vi "dl950_wave1.vi"() -> ()   [LabVIEW 2019]
uses:
  <instrlib>/Yokogawa DL950 Series/Public/Configure/Configure Module (Voltage).vi
  <instrlib>/Yokogawa DL950 Series/Public/Data/Read Waveform (Single).vi
  <instrlib>/Yokogawa DL950 Series/Yokogawa DL950 Series.lvlib
panel:
  in  "Channel (1: CH1)":u16(ring)=1 items=["", "CH1", "CH2", "CH3", "CH4", "CH5", "CH6", "CH7", "CH8", "CH9", "CH10", "CH11", "CH12", "CH13", "CH14", "CH15", "CH16"]
  in  "Vertical Coupling (1: DC)":i32(ring)=1 items=["AC", "DC", "Ground", "AC-RMS", "DC-RMS"]
  in  "Enable Calibration (F: No)":bool
  in  "Enable Auto Setup (T: Yes)":bool=TRUE
  in  "VISA resource name":refnum<visa-resource-name>
  in  "Source (1: CH1)":u16(ring)=1 items=["", "CH1", "CH2", "CH3", "CH4", "CH5", "CH6", "CH7", "CH8", "CH9", "CH10", "CH11", "CH12", "CH13", "CH14", "CH15", "CH16", "MATH1", "MATH2", "MATH3", "MATH4", "MATH5", "MATH6", "MATH7", "MATH8", "EVENT"]
  in  "Sub Channel (0: None)":i16(ring) items=["None", "SCH1", "SCH2", "SCH3", "SCH4", "SCH5", "SCH6", "SCH7", "SCH8", "SCH9", "SCH10", "SCH11", "SCH12", "SCH13", "SCH14", "SCH15", "SCH16", "SCH17", "SCH18", "SCH19", "SCH20", "SCH21", "SCH22", "SCH23", "SCH24", "SCH25", "SCH26", "SCH27", "SCH28", "SCH29", "SCH30", "SCH31", "SCH32", "SCH33", "SCH34", "SCH35", "SCH36", "SCH37", "SCH38", "SCH39", "SCH40", "SCH41", "SCH42", "SCH43", "SCH44", "SCH45", "SCH46", "SCH47", "SCH48", "SCH49", "SCH50", "SCH51", "SCH52", "SCH53", "SCH54", "SCH55", "SCH56", "SCH57", "SCH58", "SCH59", "SCH60", "SCH61", "SCH62", "SCH63", "SCH64"]
  in  "Timeout (10000 ms)":u32=10000
  out "Waveform Graph":waveform(dbl)(graph)
  in  "stop":bool
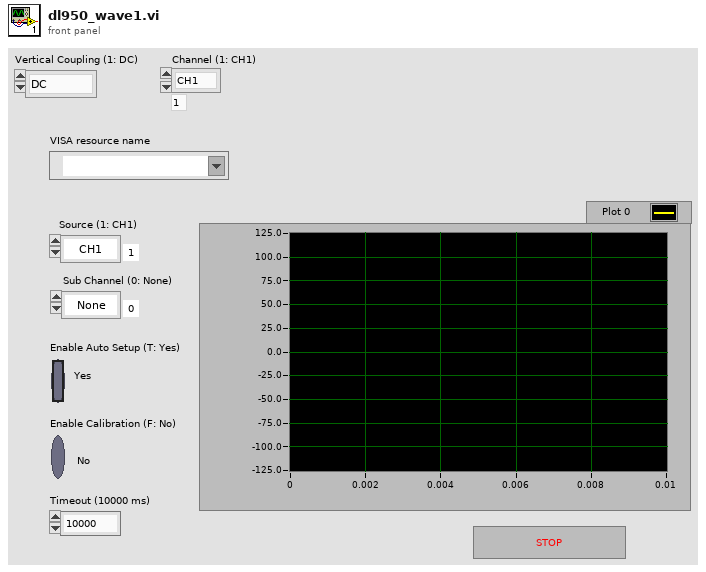
[diagram p1: front panel]
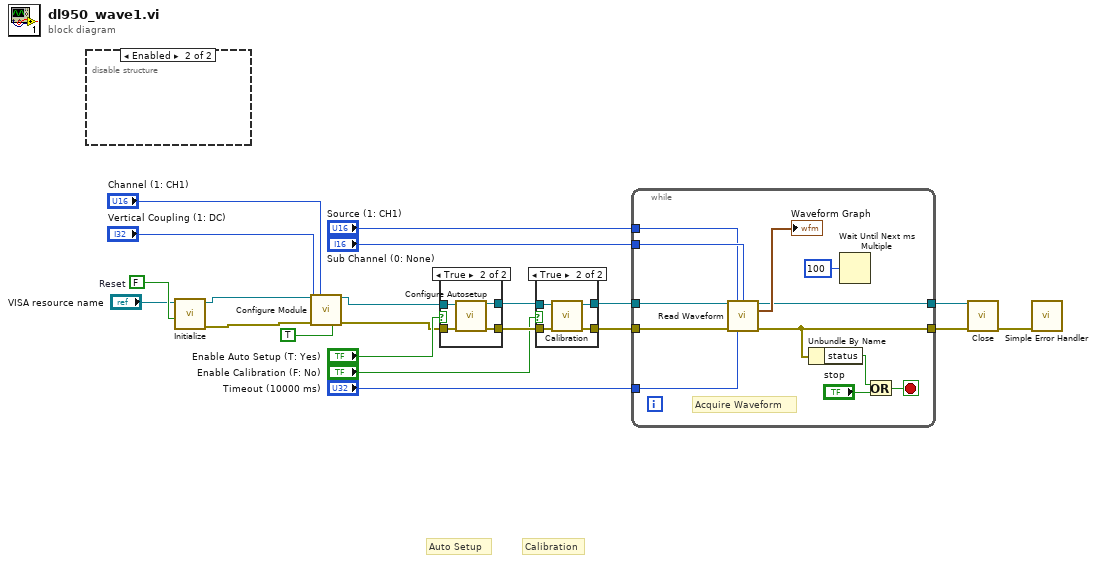
[diagram p0: block diagram]
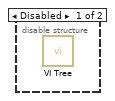
[diagram p2: hidden frame]
diagram:
  w21 = FALSE  # Reset
  # "Calibration"
  # "Auto Setup"
  n1 = disable-structure shown="Enabled" {
    frame Disabled {
      n2 = call <instrlib>:"VI Tree.vi"() -> ()  [unwired: 12 in]
    }
    frame Enabled {
    }
  }
  n3 = call <instrlib>:"Initialize.vi"("Reset (True)"=w21, "VISA resource name"="VISA resource name") -> ("error out"=w1:errorcluster, "VISA resource name out"=w2:refnum<visa-resource-name>)  [unwired: 8 in]
  n4 = call-poly <instrlib>:"Configure Module.vi"("VISA resource name"=w2, "Channel (1: CH1)"="Channel (1: CH1)", "Vertical Coupling (1: DC)"="Vertical Coupling (1: DC)", "error in (no error)"=w1, "Enable Inverted Display (F: Off)"=TRUE) -> ("VISA resource name out"=w7:refnum<visa-resource-name>, "error out"=w6:errorcluster)  [unwired: 9 in]
  n5 = case shown="True" "Enable Auto Setup (T: Yes)" {
    tunnel: w7 -> [w23 w27]
    tunnel: [w23 w26] -> w12
    tunnel: w6 -> [w22 w25]
    tunnel: [w22 w24] -> w11
    frame False {
    }
    frame True {
      n6 = call <instrlib>:"Configure Autosetup.vi"("VISA resource name"=w27, "error in (no error)"=w25) -> ("VISA resource name out"=w26:refnum<visa-resource-name>, "error out"=w24:errorcluster)  [unwired: 12 in]
    }
  }
  n7 = case shown="True" "Enable Calibration (F: No)" {
    tunnel: w12 -> [w29 w33]
    tunnel: [w29 w32] -> w10
    tunnel: w11 -> [w28 w31]
    tunnel: [w28 w30] -> w9
    frame False {
    }
    frame True {
      n8 = call <instrlib>:"Calibration.vi"("error in (no error)"=w31, "VISA resource name"=w33) -> ("error out"=w30:errorcluster, "VISA resource name out"=w32:refnum<visa-resource-name>)  [unwired: 8 in]
    }
  }
  n9 = while "Whileループ" {
    tunnel: [w39] -> w18
    tunnel: [w44] -> w19
    tunnel: w9 -> [w37]
    tunnel: w10 -> [w43]
    tunnel: "Timeout (10000 ms)" -> [w36]
    tunnel: "Sub Channel (0: None)" -> [w35]
    tunnel: "Source (1: CH1)" -> [w34]
    stop <- w40 stop-if-true
    # "Acquire Waveform"
    n10 = call-poly <instrlib>:"Read Waveform.vi"("VISA resource name"=w43, "Source (1: CH1)"=w34, "Sub Channel (0 :None)"=w35, "error in (no error)"=w37, "Timeout (10000 ms)"=w36) -> ("VISA resource name out"=w44:refnum<visa-resource-name>, "Waveform Data"=→"Waveform Graph":waveform(dbl), "error out"=w39:errorcluster)  [unwired: 8 in]
    n11 = Unbundle By Name ("名前でバンドル解除")(w39) -> ("status"=w41:bool)
    n12 = Wait Until Next ms Multiple ("次のミリ秒倍数まで待機")(millisecond multiple=u32 100) -> ()  [unwired: 1 out]
    n13 = Or(x=w41, y="stop") -> (x .or. y?=w40:bool)
  }
  n14 = call <instrlib>:"Close.vi"("error in (no error)"=w18, "VISA resource name"=w19) -> ("error out"=w20:errorcluster)  [unwired: 9 in]
  n15 = call <vilib>:"Simple Error Handler.vi"("error in (no error)"=w20) -> ()  [unwired: 4 in, 5 out]
